vi "escritura_de_I2.vi"(10 "Array 2":string[][](array[string])=[["Pi", "Li", "Lo", "Po", "E", "B", "G", "C", "I2"], ["90", "0", "0", "0", "0", "48", "0", "0", "0"]], 11 "I2\n<90,0|0,0>":bool) -> ()   [LabVIEW 2009]
uses:
  <vilib>/Utility/file.llb/Write To Spreadsheet File (string).vi
panel:
  in  "file path (dialog if empty)":path=path "C:/Users/franjas/Documents/rutinas-calibracion-slm/parametros_medida.txt"
  in  "ICImagingControl":refnum<k7>(container)
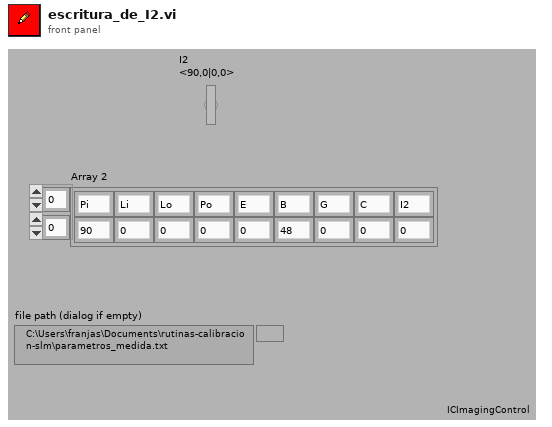
[diagram p1: front panel]
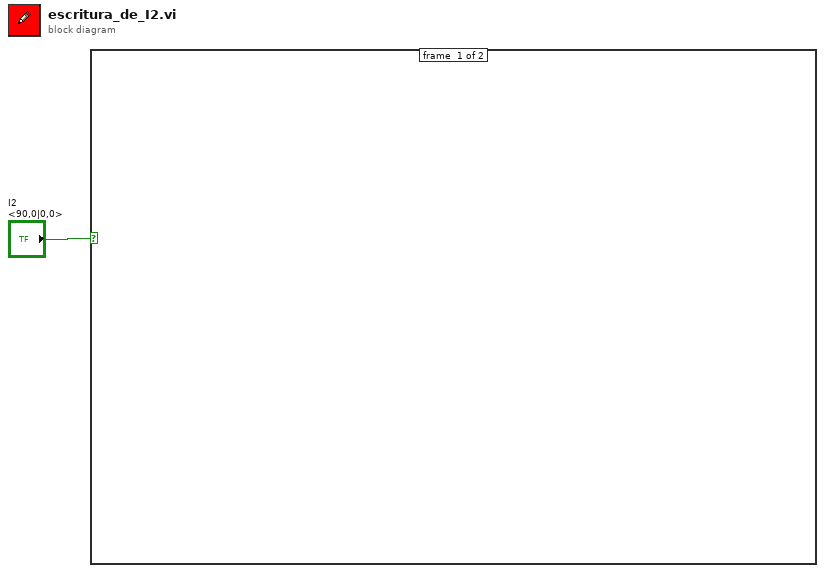
[diagram p0: block diagram]
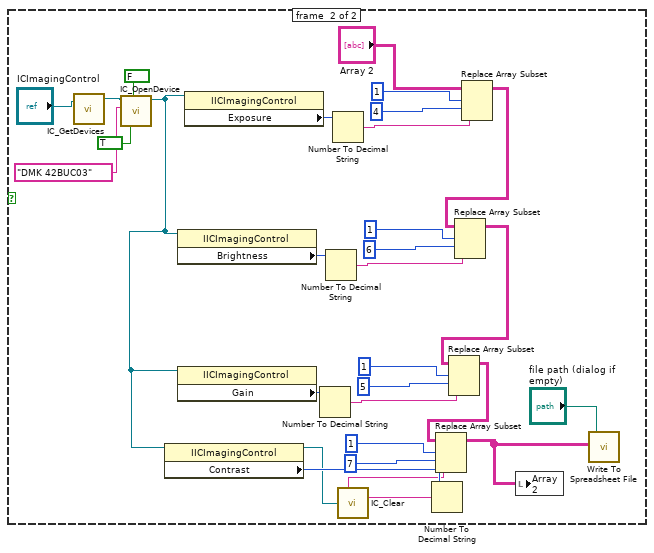
[diagram p2: hidden frame]
diagram:
  n1 = case shown="True" "I2\n<90,0|0,0>" {
    frame #0 {
    }
    frame #1 {
      n2 = call <userlib>:"IC_GetDevices.vi"("ICImagingControl In"="ICImagingControl") -> ("ICImagingControl Out"=w29:refnum<k7>)  [unwired: 1 in, 2 out]
      n3 = call <userlib>:"IC_OpenDevice.vi"("Color"=FALSE, "Live"=TRUE, "Device"="DMK 42BUC03", "ICImagingControl In"=w29) -> ("ICImagingControl Out"=w6:refnum<k7>)  [unwired: 2 in, 5 out]
      n4 = property class="IICImagingControl"(reference=w6) -> (reference out=w2:refnum<k7>, "Contrast"=w10:i32)  [unwired: 1 in, 1 out]
      n5 = property class="IICImagingControl"(reference=w6) -> ("Brightness"=w22:i32)  [unwired: 1 in, 2 out]
      n6 = property class="IICImagingControl"(reference=w6) -> ("Gain"=w18:i32)  [unwired: 1 in, 2 out]
      n7 = property class="IICImagingControl"(reference=w6) -> ("Exposure"=w26:i32)  [unwired: 1 in, 2 out]
      n8 = Number To Decimal String(number=w18) -> (decimal integer string=w15:string)  [unwired: 1 in]
      n9 = Number To Decimal String(number=w22) -> (decimal integer string=w19:string)  [unwired: 1 in]
      n10 = Number To Decimal String(number=w26) -> (decimal integer string=w23:string)  [unwired: 1 in]
      n11 = call <userlib>:"IC_Clear.vi"("ICImagingControl 2"=w2) -> ()  [unwired: 1 out]
      n12 = Number To Decimal String(number=w10) -> (decimal integer string=w7:string)  [unwired: 1 in]
      n13 = Replace Array Subset(array="Array 2", new element=w23, index (row)=1, index (col)=4 ("disabled index (col)")) -> (w12:string[][])
      n14 = Replace Array Subset(array=w12, new element=w19, index (row)=1, index (col)=6 ("disabled index (col)")) -> (w11:string[][])
      n15 = Replace Array Subset(array=w11, new element=w15, index (row)=1, index (col)=5 ("disabled index (col)")) -> (w5:string[][])
      n16 = Replace Array Subset(array=w5, new element=w7, index (row)=1, index (col)=7 ("disabled index (col)")) -> (w4:string[][])
      n17 = local write "Array 2"(w4) -> ()
      n18 = call-poly <vilib>:"Write To Spreadsheet File.vi"("2D data"=w4, "file path (dialog if empty)"="file path (dialog if empty)") -> ()  [unwired: 6 in, 1 out]
    }
  }
